vi "pmu_Check Command.vi"(8 "error in (no error)":errorcluster, 11 "command in":u16) -> (0 "error out":errorcluster, 3 "command out":u16)   [LabVIEW 2015, in "NI_EP_PMU.lvlib"]
uses:
  <vilib>/addons/Electrical Power/PMU/NI_EP_PMU.lvlib
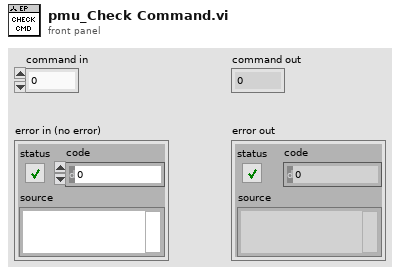
[diagram p1: front panel]
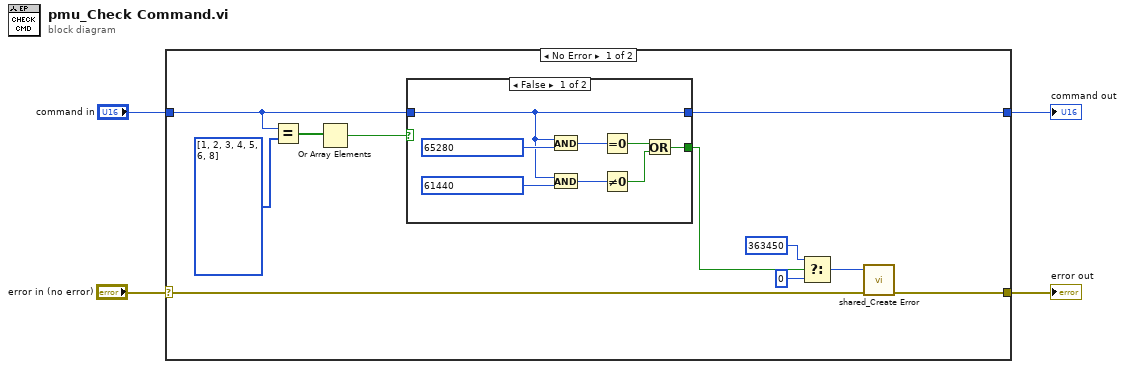
[diagram p0: block diagram]
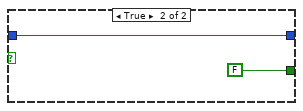
[diagram p2: hidden frame]
diagram:
  n1 = case shown="No Error" "error in (no error)" {
    selector: "error in (no error)" -> [w6 w26]
    tunnel: "command in" -> [w15 _]
    tunnel: [w14 _] -> w3
    tunnel: [w5 w26] -> w1
    frame No Error {
      n2 = Equal?(x=w15, y=u16[] [1, 2, 3, 4, 5, 6, 8]) -> (x = y?=w11:bool[])
      n3 = Or Array Elements(Boolean array=w11) -> (logical OR=w10:bool)
      n4 = case shown="False" w10 {
        tunnel: w15 -> [w16 w24]
        tunnel: [w17 FALSE ("result")] -> w13
        tunnel: [w16 w24] -> w14
        frame False {
          n5 = And(x=w16, y=u16 65280 ("Command")) -> (x .and. y?=w22:u16)
          n6 = And(x=w16, y=u16 61440 ("Command")) -> (x .and. y?=w20:u16)
          n7 = Equal To 0?(x=w22) -> (x = 0?=w19:bool)
          n8 = Not Equal To 0?(x=w20) -> (x != 0?=w18:bool)
          n9 = Or(x=w19, y=w18) -> (x .or. y?=w17:bool)
        }
        frame True {
        }
      }
      n10 = Select(t=363450 ("error code (0)"), s=w13, f=0 ("error code (0)")) -> (s? t:f=w7:i32)
      n11 = call <vilib>:"shared_Create Error.vi"("error in (no error)"=w6, "error code (0)"=w7) -> ("error out"=w5:errorcluster)  [unwired: 9 in]
    }
    frame Error {
    }
  }
  "command out" <- w3
  "error out" <- w1
